vi "Initialize.vi"(8 "error in (no error)":errorcluster, 9 "Requestor":string, 10 "Requestee":string, 11 "Mag Lab TIMER in":refnum<class "Measurement Timer.lvclass">) -> (0 "error out":errorcluster, 3 "Mag Lab TIMER out":refnum<class "Measurement Timer.lvclass">)   [LabVIEW 2015, in "Measurement Timer.lvclass"]
uses:
  Measurement Timer.lvclass
  Measurement Timer.lvclass/Measurement Timer.ctl
  Mag Lab Measurement/Mag Lab Measurement.lvclass
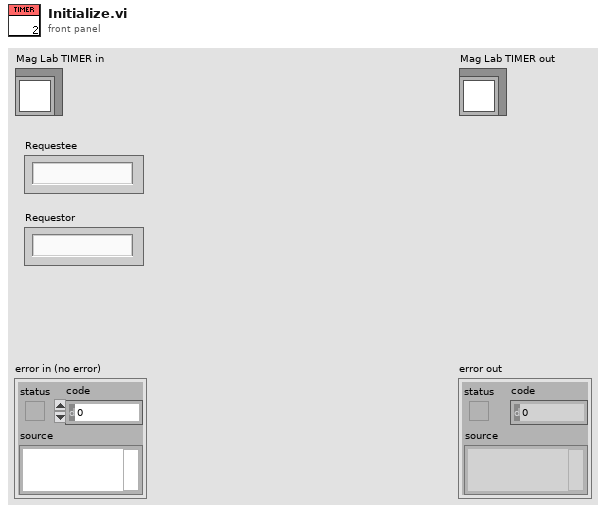
[diagram p1: front panel]
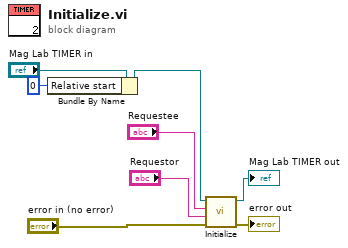
[diagram p0: block diagram]
diagram:
  n1 = Bundle By Name(cluster="Mag Lab TIMER in", "Relative start"=u64 0) -> (w2:refnum<class "Measurement Timer.lvclass">)
  n2 = call-parent "Initialize.vi"("error in (no error)"="error in (no error)", "Requestor"="Requestor", "Requestee"="Requestee", "Mag Lab Hardware in"=w2) -> ("error out"=→"error out":errorcluster, "Mag Lab Hardware out"=→"Mag Lab TIMER out":refnum<class "Measurement Timer.lvclass">)  [unwired: 6 in]
